vi "zadanie_3.vi"() -> ()   [LabVIEW 2020]
panel:
  in  "?":enum32{"Sinus", "Prostokąt", "Piłokształtny"}(tab)
  in  "częstotliwość\n[Hz]":dbl(slide) scale=0.0..100.0
  out "?":dynamicdata(graph)
  out "?":dynamicdata(graph)
  in  "częstotliwość\n[Hz]":dbl(slide) scale=0.0..100.0
  out "?":dynamicdata(graph)
  in  "częstotliwość\n[Hz]":dbl(slide) scale=0.0..100.0
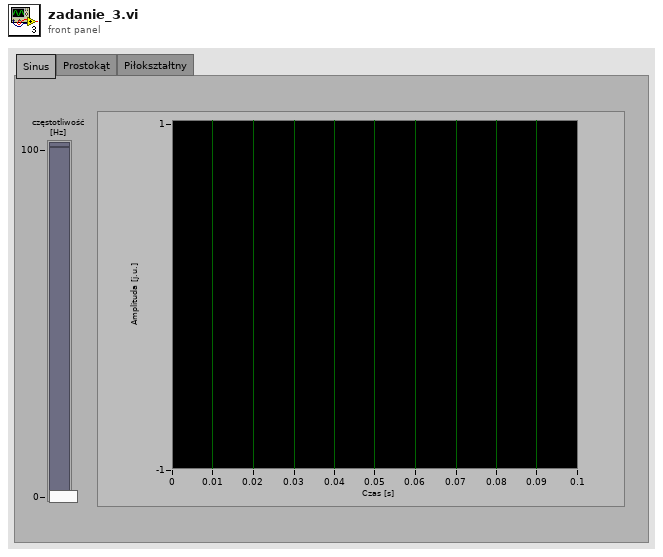
[diagram p1: front panel]
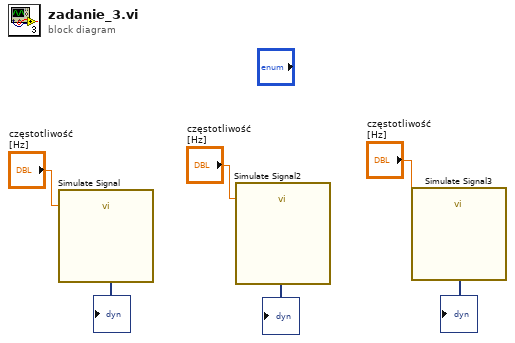
[diagram p0: block diagram]
diagram:
  n1 = call "Simulate Signal"("Frequency"="częstotliwość\n[Hz]") -> ("Sine"=→"?":dynamicdata)  [unwired: 13 in, 1 out]
  n2 = call "Simulate Signal2"("Frequency"="częstotliwość\n[Hz]") -> ("Square"=→"?":dynamicdata)  [unwired: 13 in, 1 out]
  n3 = call "Simulate Signal3"("Frequency"="częstotliwość\n[Hz]") -> ("Sawtooth"=→"?":dynamicdata)  [unwired: 13 in, 1 out]
